vi "ABM Verificacion Project.vi"() -> ()   [LabVIEW 2010]
panel:
  out "?":string
  in  "Assambled by":string
  in  "Serial Number":string
  # "ABM Verification Software For ABM Assembling Line"
  # "ABM Serial Numbre"
  # "Assembled by"
  # "Assembled Date"
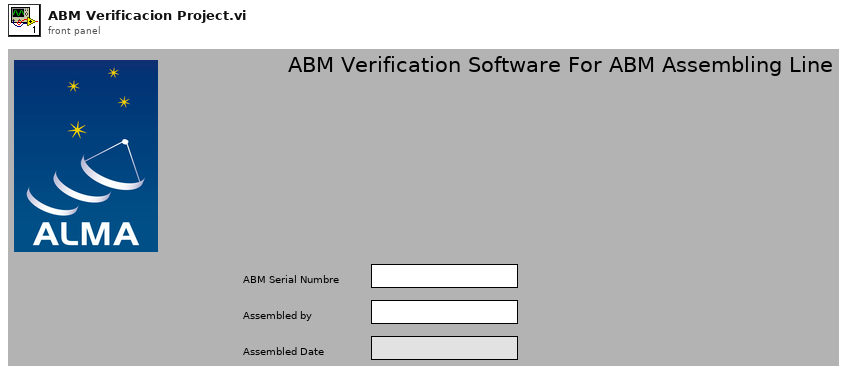
[diagram p1: front panel]
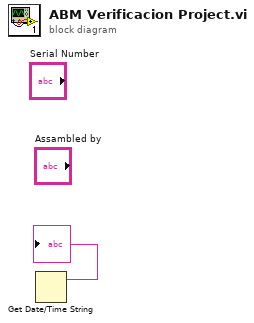
[diagram p0: block diagram]
diagram:
  n1 = Get Date/Time String() -> (date string=→"?":string)  [unwired: 3 in, 1 out]
